vi "ViewContact.vi"(7 "LabVIEW Web Service Request":refnum<class "Web Request.lvclass">, 10 "Edit":bool, 11 "ID":u32) -> ()   [LabVIEW 2014]
doc: "This HTTP Method VI shows an existing contact and optionally provides a form for editing the contact information."
uses:
  <vilib>/wsapi/Web Request.lvclass
  <vilib>/wsapi/class/subVIs/Set String ESP Variable.vi
  Libraries/Contact Data/Contact Data.lvlib
panel:
  # "Because this is an HTTP Method VI, LabVIEW Web Service Request is populated automatically."
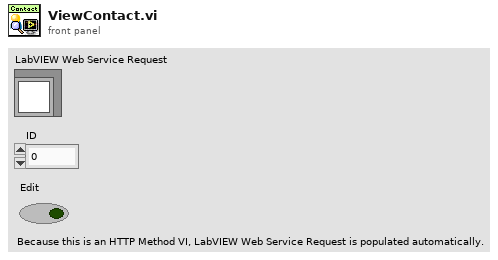
[diagram p1: front panel]
types:
  T1 = typedef "Contact Data.lvlib/Contact.ctl" = cluster{"ID":u32, "UUID":string, "Name":string, "Iteration":i32, "Posit Array":T2[], "Controls":T3, "DestArray":T4[], "SetSpeed":dbl, "Speed":dbl}
  T2 = typedef "Contact Data.lvlib/Position.ctl" = cluster{"X":dbl, "Y":dbl, "Z":dbl}
  T3 = typedef "Contact Data.lvlib/Controls.ctl" = cluster{"throttle":dbl, "brake":dbl, "horn":dbl, "wait":dbl}
  T4 = typedef "Contact Data.lvlib/DestinationCluster.ctl" = cluster{"Desination":string, "DestControls":T5, "Timer":u32, "Set Timer":u32, "Time Stamp":timestamp, "Repeat?":bool, "Optional Data":string, "Distance":dbl}
  T5 = typedef "Contact Data.lvlib/DesinationControls.ctl" = enum16{"Tracker", "Manual", "Stop", "Station DateTime", "Station Timer", "Maintain"}
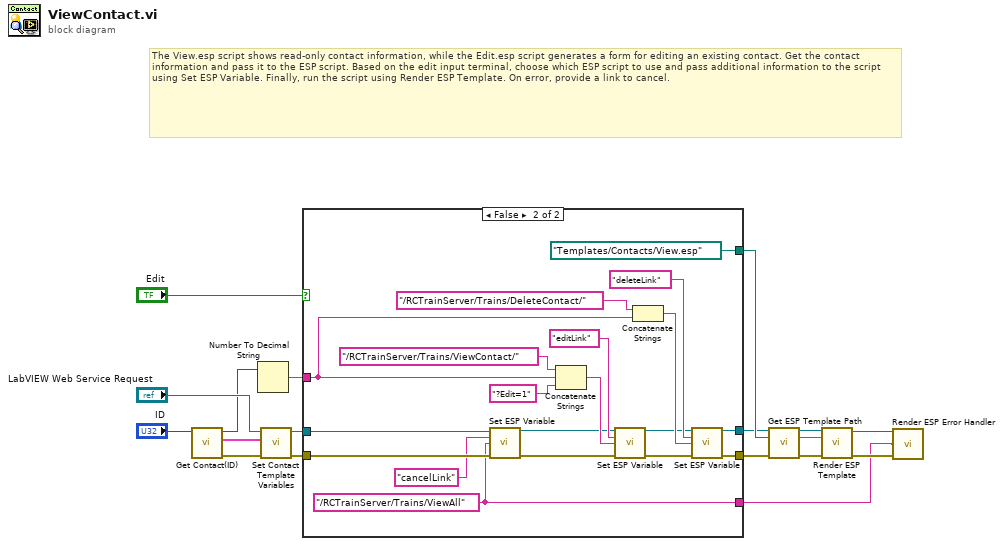
[diagram p0: block diagram]
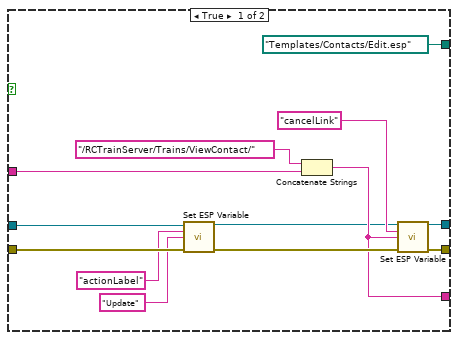
[diagram p2: hidden frame]
diagram:
  # "The View.esp script shows read-only contact information, while the Edit.esp script generates a form for editing an existing contact. Get the contact information and pass it to the ESP script. Based on the edit input terminal, choose which ESP script to use and pass additional information to the script using Set ESP Variable. Finally, run the script using Render ESP Template. On error, provide a link to cancel."
  n1 = call "Get Contact(ID).vi"("ID"="ID") -> ("error out"=w4:errorcluster, "Contact"=w5:T1, "ID dup"=w6:u32)  [unwired: 8 in]
  n2 = Number To Decimal String(number=w6) -> (decimal integer string=w17:string)  [unwired: 1 in]
  n3 = call "Set Contact Template Variables.vi"("error in (no error)"=w4, "Contact"=w5, "LabVIEW Web Service Request"="LabVIEW Web Service Request") -> ("error out"=w15:errorcluster, "LabVIEW Web Service Request out"=w14:refnum<class "Web Request.lvclass">)  [unwired: 7 in]
  n4 = case shown="False" "Edit" {
    tunnel: [path "Templates/Contacts/Edit.esp" path "Templates/Contacts/View.esp"] -> w13
    tunnel: w14 -> [w19 w33]
    tunnel: w15 -> [w31 w50]
    tunnel: [w27 w45] -> w1
    tunnel: [w26 w44] -> w12
    tunnel: w17 -> [w23 w38]
    tunnel: [w21 w36] -> w3
    frame True {
      n5 = call-poly <vilib>:"Set ESP Variable.vi"("LabVIEW Web Service Request"=w19, "key"="actionLabel", "value"="Update", "error in (no error)"=w31) -> ("LabVIEW Web Service Request out"=w20:refnum<class "Web Request.lvclass">, "error out"=w28:errorcluster)  [unwired: 10 in]
      n6 = Concatenate Strings("/RCTrainServer/Trains/ViewContact/" ("value"), w23) -> (w21:string)
      n7 = call-poly <vilib>:"Set ESP Variable.vi"("LabVIEW Web Service Request"=w20, "key"="cancelLink", "value"=w21, "error in (no error)"=w28) -> ("LabVIEW Web Service Request out"=w27:refnum<class "Web Request.lvclass">, "error out"=w26:errorcluster)  [unwired: 10 in]
    }
    frame False {
      w36 = "/RCTrainServer/Trains/ViewAll" ("value")
      n8 = call-poly <vilib>:"Set ESP Variable.vi"("LabVIEW Web Service Request"=w33, "key"="cancelLink", "value"=w36, "error in (no error)"=w50) -> ("LabVIEW Web Service Request out"=w34:refnum<class "Web Request.lvclass">, "error out"=w48:errorcluster)  [unwired: 10 in]
      n9 = Concatenate Strings("/RCTrainServer/Trains/ViewContact/" ("value"), w38, "?Edit=1" ("string")) -> (w39:string)
      n10 = call-poly <vilib>:"Set ESP Variable.vi"("LabVIEW Web Service Request"=w34, "key"="editLink", "value"=w39, "error in (no error)"=w48) -> ("LabVIEW Web Service Request out"=w32:refnum<class "Web Request.lvclass">, "error out"=w46:errorcluster)  [unwired: 10 in]
      n11 = Concatenate Strings("/RCTrainServer/Trains/DeleteContact/" ("value"), w38) -> (w40:string)
      n12 = call-poly <vilib>:"Set ESP Variable.vi"("LabVIEW Web Service Request"=w32, "key"="deleteLink", "value"=w40, "error in (no error)"=w46) -> ("LabVIEW Web Service Request out"=w45:refnum<class "Web Request.lvclass">, "error out"=w44:errorcluster)  [unwired: 10 in]
    }
  }
  n13 = call "Get ESP Template Path.vi"("LabVIEW Web Service Request"=w1, "Relative Template Path"=w13, "error in (no error)"=w12) -> ("LabVIEW Web Service Request out"=w2:refnum<class "Web Request.lvclass">, "Template Name"=w8:string, "error out"=w11:errorcluster)  [unwired: 10 in]
  n14 = call <vilib>:"Render ESP Template.vi"("LabVIEW Web Service Request"=w2, "espName"=w8, "error in (no error)"=w11) -> ("LabVIEW Web Service Request out"=w9:refnum<class "Web Request.lvclass">, "error out"=w10:errorcluster)  [unwired: 11 in]
  n15 = call "Render ESP Error Handler.vi"("LabVIEW Web Service Request"=w9, "Link"=w3, "error in (no error)"=w10) -> ()  [unwired: 11 in, 2 out]
